vi "Set Force.vi"(8 "error in (no error)":errorcluster, 10 "force (V)":dbl, 11 "Force Sensor in":refnum<class "Force Sensor.lvclass">) -> (0 "error out":errorcluster, 3 "Force Sensor out":refnum<class "Force Sensor.lvclass">)   [LabVIEW 2020, in "Force Sensor.lvclass"]
uses:
  Force Sensor.lvclass
  Force Sensor.lvclass/Force Sensor.ctl
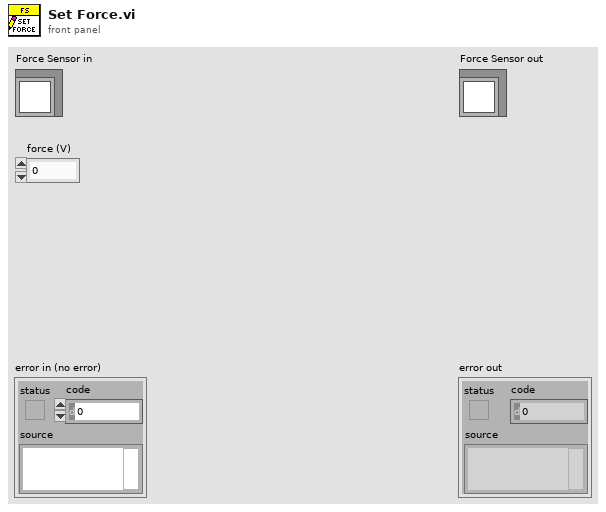
[diagram p1: front panel]
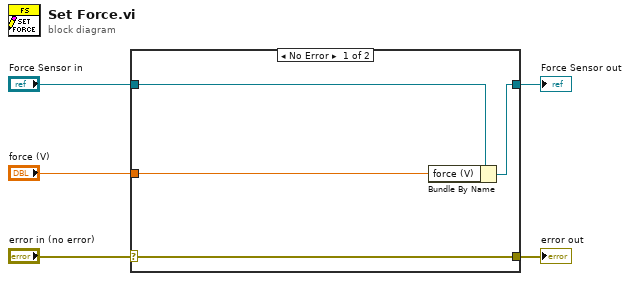
[diagram p0: block diagram]
diagram:
  n1 = case shown="No Error" "error in (no error)" {
    selector: "error in (no error)" -> [w9 w10]
    tunnel: [w9 w10] -> w4
    tunnel: [w7 w11] -> w2
    tunnel: "Force Sensor in" -> [w8 w11]
    tunnel: "force (V)" -> [w6 _]
    frame No Error {
      n2 = Bundle By Name(cluster=w8, "force (V)"=w6) -> (w7:refnum<class "Force Sensor.lvclass">)
    }
    frame Error {
    }
  }
  "error out" <- w4
  "Force Sensor out" <- w2
